vi "nanocal-frontend-tcplink-server.vi"() -> ()   [LabVIEW 2020]
doc: "Demonstrates how to set up a basic TCP connection, send data to the specified port once a connection has been established, and terminate the connection once the data has been sent. This VI is designed to stop if the TCP connection is terminated. The data sent in this example is an array of random numbers."
uses:
  icicle.ctl
  publisher action.ctl
panel:
  in  "Tab Control":enum32{"Page 1", "Page 2"}(tab)
  in  "Stop":bool
  in  "port":u16=6340
  in  "timeout (ms)":i32=30000
  in  "wait (ms)":u32=50
  out "nanocal data":T1[](array[typedef])=[{"name"="frequency", "units"="Hz", "data"=22.99998355490133}, {"name"="Cs/T", "units"="J/K^2", "data"=3.886931203146552e-15}, {"name"="Ts", "units"="K", "data"=0.008240058514617926}, {"name"="Ts^2", "units"="K^2", "data"=6.789856432432739e-05}, {"name"="Tr", "units"="K", "data"=0.01160124820696135}, {"name"="Cs", "units"="J/K", "data"=3.2028540556221847e-17}, {"name"="Cr", "units"="J/K", "data"=-7.008174377596114e-24}, {"name"="Ks", "units"="W/K", "data"=1.2438486299100949e-14}, {"name"="Kr", "units"="W/K", "data"=1.6481186390496327e-21}, {"name"="Rs-therm", "units"="Ohm", "data"=284324.59659854736}, {"name"="Rr-therm", "units"="Ohm", "data"=88760.8838737066}, {"name"="Cr/T", "units"="J/K^2", "data"=-6.040879612756536e-22}, {"name"="dlogR/dlogT -- S ", "units"="a.u.", "data"=inf}, {"name"="tau", "units"="s", "data"=0.0025749548446692312}, {"name"="tan(phi)", "units"="a.u", "data"=0.7442297164193036}, {"name"="Ts,ac", "units"="K", "data"=0.0}, {"name"="Tr,ac", "units"="K", "data"=0.014181653003783065}, {"name"="Hs,ac,out", "units"="V", "data"=0.0}, {"name"="Offset,dc,out", "units"="V", "data"=1.0000000009313226}, {"name"="Vdiff,ac", "units"="V", "data"=4.514115240142335e-09}, {"name"="Vdiff,ac,phase", "units"="deg", "data"=22.78519616358481}, {"name"="Stherm,ac,out", "units"="V", "data"=0.0}, {"name"="Rtherm,ac,out", "units"="V", "data"=0.0}, {"name"="CV1 -- Re", "units"="V", "data"=4.161848337012954e-09}, {"name"="CV1 -- Im", "units"="V", "data"=1.7482147525369406e-09}, {"name"="DV2 -- Re", "units"="V", "data"=4.7405574273041075e-09}, {"name"="DV2 -- Im", "units"="V", "data"=-1.6949847562010464e-08}, {"name"="AV2 -- Re", "units"="V", "data"=8.192959885292162e-10}, {"name"="AV2 -- Im", "units"="V", "data"=1.2099754860062243e-09}, {"name"="Vdiff,norm, Re", "units"="V", "data"=1.307901931118997e+18}, {"name"="Vdiff,norm, Im", "units"="V", "data"=5.4939374664835776e+17}, {"name"="Resistance.RHr", "units"="ohm", "data"=110502.77415660422}, {"name"="Resistance.RHs", "units"="ohm", "data"=149199.95763357717}]
  # "nanocal tcplink -- Server"
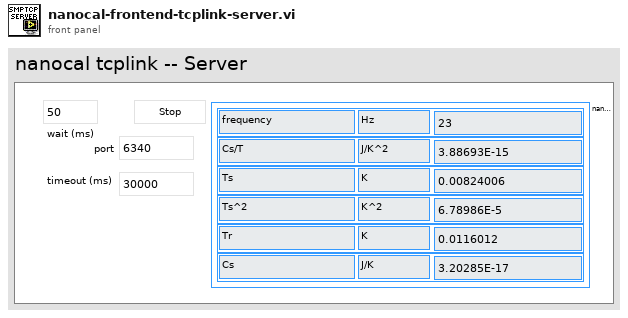
[diagram p1: front panel]
types:
  T1 = typedef "icicle.ctl" = cluster{"name":string, "units":string, "data":dbl}
  T2 = typedef "publisher action.ctl" = enum16{"set", "get", "init", "check"}
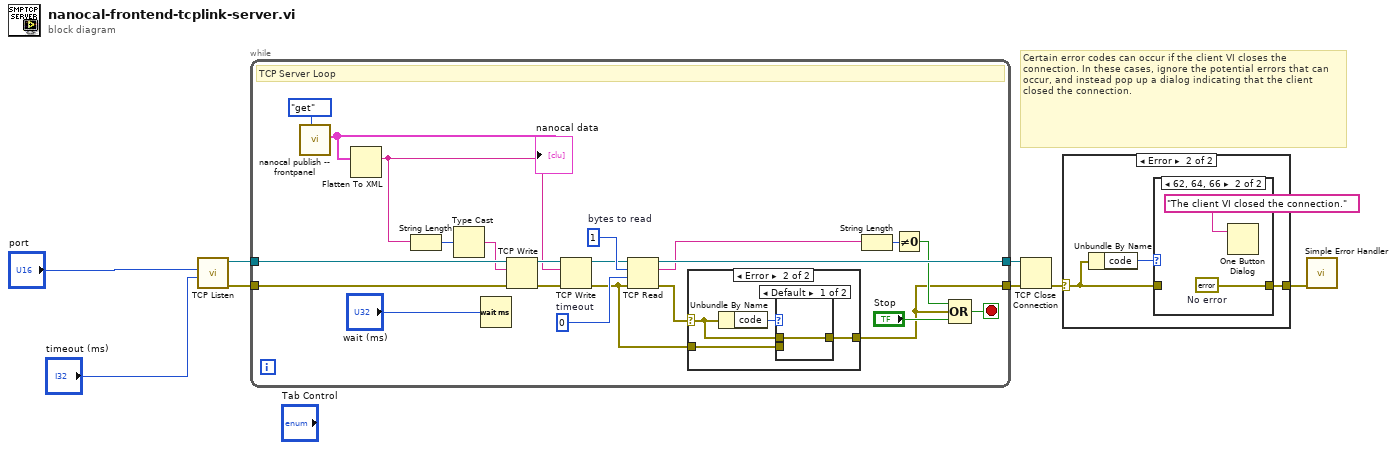
[diagram p0: block diagram]
diagram:
  # "Certain error codes can occur if the client VI closes the connection. In these cases, ignore the potential errors that can occur, and instead pop up a dialog indicating that the client closed the connection."
  n1 = call <vilib>:"TCP Listen.vi"("timeout ms (wait forever: -1)"="timeout (ms)", "port"="port") -> ("error out"=w3:errorcluster, "connection ID"=w4:refnum<k5>)  [unwired: 5 in, 3 out]
  n2 = while {
    tunnel: [w13] -> w7
    tunnel: [w19] -> w8
    tunnel: w4 -> [w30]
    tunnel: w3 -> [w23]
    stop <- w24 stop-if-true
    w18 = 0  # timeout
    w21 = 1  # bytes to read
    # "TCP Server Loop"
    n3 = call "nanocal publish -- frontpanel.vi"("publisher action"=publisher_action."get") -> ("nanocal data array OUT"=w10:T1[])  [unwired: 10 in]
    "nanocal data" <- w10
    n4 = Flatten To XML(6:w10) -> (2:w9:string)
    n5 = String Length(string=w9) -> (length=w27:i32)
    n6 = Type Cast(x=w27) -> (*(type *) &x=w26:string)  [unwired: 1 out]
    n7 = Wait (ms)(milliseconds to wait="wait (ms)") -> ()  [unwired: 1 out]
    n8 = TCP Write(connection ID=w30, data in=w26, error in (no error)=w23) -> (connection ID out=w29:refnum<k5>, error out=w28:errorcluster)  [unwired: 2 out]
    n9 = TCP Write(connection ID=w29, data in=w9, error in (no error)=w28) -> (connection ID out=w20:refnum<k5>, error out=w12:errorcluster)  [unwired: 2 out]
    n10 = TCP Read(connection ID=w20, bytes to read=w21, error in (no error)=w12, 9:w18) -> (connection ID out=w19:refnum<k5>, data out=w16:string, error out=w14:errorcluster)  [unwired: 1 out]
    n11 = case shown="Error" w14 {
      selector: w14 -> [w31 w34]
      tunnel: [w31 w32] -> w13
      tunnel: w12 -> [_ w33]
      frame No Error {
      }
      frame Error {
        n12 = Unbundle By Name(w34) -> ("code"=w35:i32)
        n13 = case shown="Default" w35 {
          tunnel: w34 -> [w36 _]
          tunnel: w33 -> [_ w37]
          tunnel: [w36 w37] -> w32
          frame Default {
          }
          frame 56 {
          }
        }
      }
    }
    n14 = String Length(string=w16) -> (length=w17:i32)
    n15 = Not Equal To 0?(x=w17) -> (x != 0?=w15:bool)
    n16 = Compound Arithmetic op=OR(w15, w13, "Stop") -> (w24:bool)
  }
  n17 = TCP Close Connection(connection ID=w8, error in (no error)=w7) -> (error out=w6:errorcluster)  [unwired: 2 out]
  n18 = case shown="Error" w6 {
    selector: w6 -> [w38 w40]
    tunnel: [w38 w39] -> w5
    frame No Error {
    }
    frame Error {
      n19 = Unbundle By Name(w40) -> ("code"=w41:i32)
      n20 = case shown="62, 64, 66" w41 {
        tunnel: w40 -> [w42 _]
        tunnel: [w42 w44] -> w39
        frame Default {
        }
        frame 62, 64, 66 {
          w44 = errorcluster {"status"=FALSE, "code"=0, "source"=""}  # No error
          n21 = One Button Dialog(message="The client VI closed the connection." ("Client Closed")) -> ()  [unwired: 1 in, 1 out]
        }
      }
    }
  }
  n22 = call <vilib>:"Simple Error Handler.vi"("error in (no error)"=w5) -> ()  [unwired: 1 in, 8 out]
